vi "imaq save GEECS.vi"(7 "Status":T2, 8 "error in (no error)":errorcluster, 9 "file already written":bool, 10 "Refnum in":T1, 11 "FakeCamera in":refnum<class "Point Grey Camera.lvclass">) -> (0 "error out":errorcluster, 3 "FakeCamera out":refnum<class "Point Grey Camera.lvclass">)   [LabVIEW 2020, in "Point Grey Camera.lvclass"]
uses:
  Point Grey Camera.lvclass
  Image save type.ctl
  1st or last shot of scan.ctl
  IMAQ Image.ctl
  Point Grey Camera.lvclass/Point Grey Camera.ctl
panel:
  out "Save type":T3
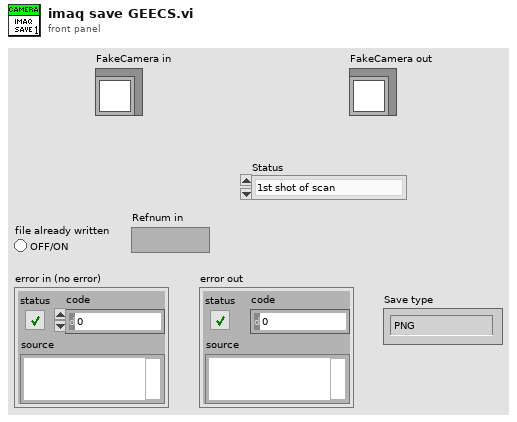
[diagram p1: front panel]
types:
  T1 = typedef "IMAQ Image.ctl" = refnum<image>
  T2 = typedef "1st or last shot of scan.ctl" = enum16{"1st shot of scan", "1st shot after scan end", "other"}
  T3 = typedef "Image save type.ctl" = enum16{"PNG", "BMP", "JPEG", "TDMS", "hdf5"}
  T4 = typedef "OnOffTypeDef.ctl" = enum16{"off", "on"}
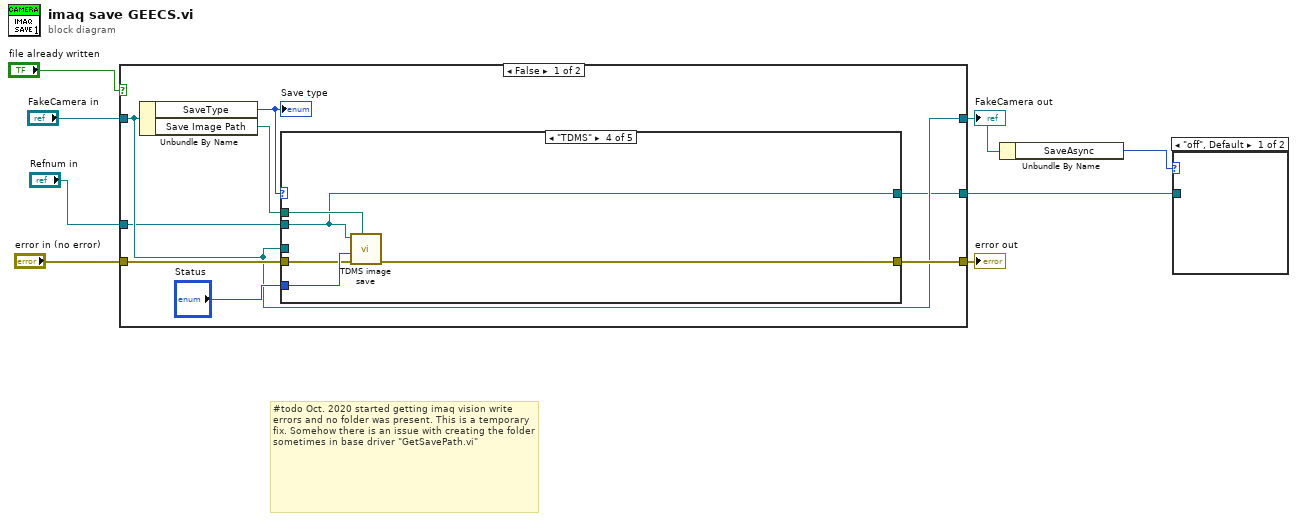
[diagram p0: block diagram]
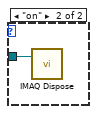
[diagram p2: hidden frame]
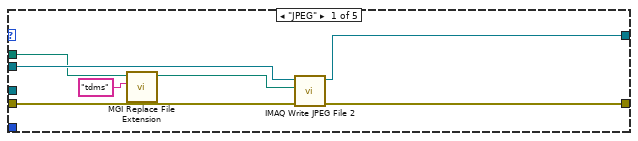
[diagram p3: hidden frame]
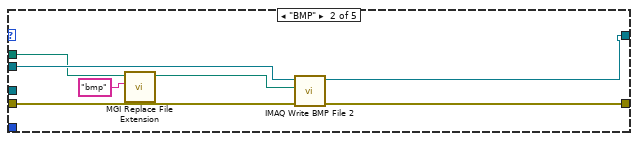
[diagram p4: hidden frame]
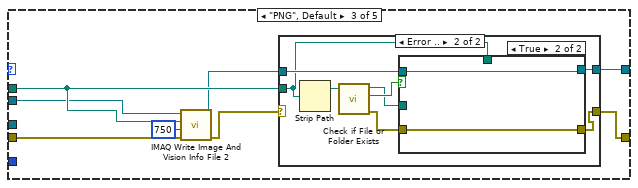
[diagram p5: hidden frame]
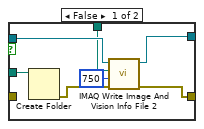
[diagram p7: hidden frame]
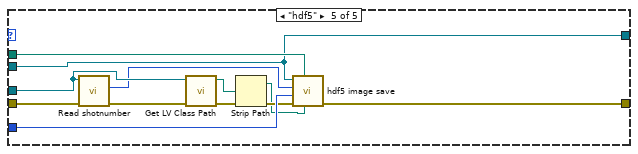
[diagram p8: hidden frame]
diagram:
  # "#todo Oct. 2020 started getting imaq vision write errors and no folder was present. This is a temporary fix. Somehow there is an issue with creating the folder sometimes in base driver \"GetSavePath.vi\""
  n1 = case shown="False" "file already written" {
    tunnel: [w16 w76] -> w8
    tunnel: "error in (no error)" -> [w12 w76]
    tunnel: [w11 w75] -> w2
    tunnel: "FakeCamera in" -> [w11 w75]
    tunnel: [w10 w74] -> w4
    tunnel: "Refnum in" -> [w9 w74]
    frame False {
      n2 = Unbundle By Name(w11) -> ("SaveType"=w13:T3, "Save Image Path"=w15:path)
      "Save type" <- w13
      n3 = case shown="\"TDMS\"" w13 {
        tunnel: w12 -> [w23 w30 w38 w59 w68]
        tunnel: w9 -> [w21 w28 w33 w58 w63]
        tunnel: w15 -> [w18 w26 w34 w62 w73]
        tunnel: [w20 w25 w35 w61 w72] -> w16
        tunnel: "Status" -> [_ _ _ w60 w71]
        tunnel: w11 -> [_ _ _ _ w69]
        tunnel: [w17 w24 w32 w58 w63] -> w10
        frame "JPEG" {
          n4 = call "MGI Replace File Extension.vi"("New Extension (txt)"="tdms", "Path In"=w18) -> ("Path Out"=w22:path)  [unwired: 8 in, 1 out]
          n5 = call "IMAQ Write JPEG File 2"("error in (no error)"=w23, "File Path"=w22, "Image"=w21) -> ("error out"=w20:errorcluster, "Image Out (duplicate)"=w17:T1)  [unwired: 7 in]
        }
        frame "BMP" {
          n6 = call "MGI Replace File Extension.vi"("New Extension (txt)"="bmp", "Path In"=w26) -> ("Path Out"=w29:path)  [unwired: 8 in, 1 out]
          n7 = call "IMAQ Write BMP File 2"("error in (no error)"=w30, "File Path"=w29, "Image"=w28) -> ("error out"=w25:errorcluster, "Image Out (duplicate)"=w24:T1)  [unwired: 7 in]
        }
        frame "PNG", Default {
          n8 = call "IMAQ Write Image And Vision Info File 2"("error in (no error)"=w38, "Image Quality"=u32 750, "File Path"=w34, "Image"=w33) -> ("error out"=w36:errorcluster, "Image Out (duplicate)"=w31:T1)  [unwired: 6 in]
          n9 = case shown="Error .." w36 {
            selector: w36 -> [w40 _]
            tunnel: [w40 w43] -> w35
            tunnel: w34 -> [_ w42]
            tunnel: w31 -> [w39 w44]
            tunnel: [w39 w41] -> w32
            frame No Error {
            }
            frame Error {
              n10 = Strip Path(path=w42) -> (stripped path=w48:path)  [unwired: 1 out]
              n11 = call "Check if File or Folder Exists.vi"("path"=w48) -> ("error out"=w45:errorcluster, "file or folder exists?"=w47:bool, "dup path"=w46:path)  [unwired: 1 in, 7 out]
              n12 = case shown="True" w47 {
                tunnel: w46 -> [w55 _]
                tunnel: [w51 w57] -> w43
                tunnel: w45 -> [_ w57]
                tunnel: w44 -> [w53 w56]
                tunnel: w42 -> [w50 _]
                tunnel: [w49 w56] -> w41
                frame False {
                  n13 = Create Folder(path (use dialog)=w55) -> (error out=w52:errorcluster)  [unwired: 1 in, 3 out]
                  n14 = call "IMAQ Write Image And Vision Info File 2"("error in (no error)"=w52, "Image Quality"=u32 750, "File Path"=w50, "Image"=w53) -> ("error out"=w51:errorcluster, "Image Out (duplicate)"=w49:T1)  [unwired: 6 in]
                }
                frame True {
                }
              }
            }
          }
        }
        frame "TDMS" {
          n15 = call "TDMS image save.vi"("Save Image Path"=w62, "error in (no error)"=w59, "Status"=w60, "Refnum in"=w58) -> ("error out"=w61:errorcluster)  [unwired: 7 in]
        }
        frame "hdf5" {
          n16 = call-dynamic "Read shotnumber.vi"("error in (no error)"=w68, "BaseDriver in"=w69) -> ("error out"=w66:errorcluster, "shotnumber"=w67:i32)  [unwired: 6 in, 2 out]
          n17 = call "Get LV Class Path.vi"("error in (no error)"=w66, "object"=w69) -> ("error out"=w70:errorcluster, "class path"=w65:path)  [unwired: 8 in]
          n18 = Strip Path(path=w65) -> (stripped path=w64:path)  [unwired: 1 out]
          n19 = call "hdf5 image save.vi"("class path"=w64, "Save Image Path"=w73, "error in (no error)"=w70, "Status"=w71, "image #"=w67, "Refnum in"=w63) -> ("error out"=w72:errorcluster)  [unwired: 5 in]
        }
      }
    }
    frame True {
    }
  }
  "error out" <- w8
  "FakeCamera out" <- w2
  n20 = Unbundle By Name(w2) -> ("SaveAsync"=w1:T4)
  n21 = case shown="\"off\", Default" w1 {
    tunnel: w4 -> [_ w77]
    frame "off", Default {
    }
    frame "on" {
      n22 = call "IMAQ Dispose"("Image"=w77) -> ()  [unwired: 5 in, 1 out]
    }
  }
